vi "connect socket.vi"(8 "error in (no error)":errorcluster, 11 "Socket in":refnum<class "Socket2.lvclass">) -> (0 "error out":errorcluster, 3 "Socket out":refnum<class "Socket2.lvclass">)   [LabVIEW 2018, in "Socket2.lvclass"]
uses:
  Socket2.lvclass
  Socket2.lvclass/Socket2.ctl
  <vilib>/addons/zeromq/zmq_socket.lvclass
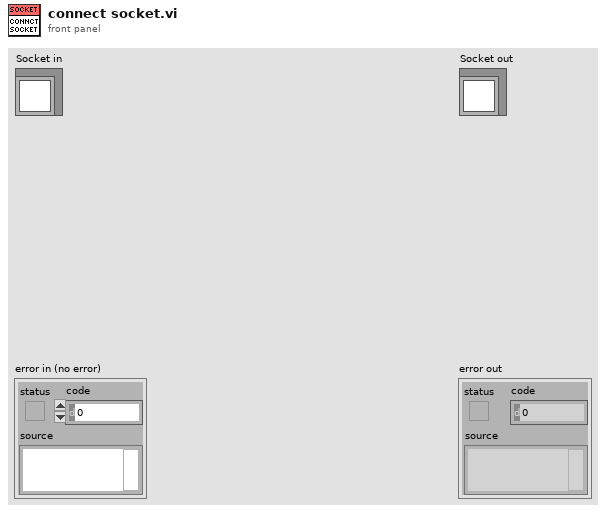
[diagram p1: front panel]
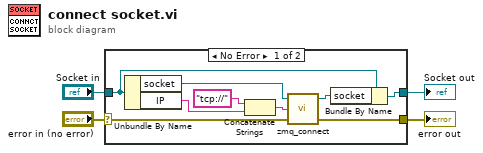
[diagram p0: block diagram]
diagram:
  n1 = case shown="No Error" "error in (no error)" {
    selector: "error in (no error)" -> [w13 w15]
    tunnel: [w12 w15] -> w3
    tunnel: [w9 w14] -> w1
    tunnel: "Socket in" -> [w10 w14]
    frame No Error {
      n2 = Unbundle By Name(w10) -> ("socket"=w11:refnum<class "zmq_socket.lvclass">, "IP"=w7:string)
      n3 = Concatenate Strings("tcp://" ("string"), w7) -> (w6:string)
      n4 = call <vilib>:"zmq_connect.vi"("error in"=w13, "endpoint"=w6, "socket in"=w11) -> ("error out"=w12:errorcluster, "socket out"=w8:refnum<class "zmq_socket.lvclass">)  [unwired: 1 in]
      n5 = Bundle By Name(cluster=w10, "socket"=w8) -> (w9:refnum<class "Socket2.lvclass">)
    }
    frame Error {
    }
  }
  "error out" <- w3
  "Socket out" <- w1
